vi "D - Level HWEng Port with Power Meter.vi"(5 "PM Ref":T1, 7 "Port (Port 3)":enum16{"Port 3", "Port 1(1)", "Port 1(2)"}(ring), 8 "error in (no error)":errorcluster, 9 "Frequency, MHz":dbl format="%.2f", 10 "Target Power, dBm":dbl format="%.2f") -> (0 "error out":errorcluster, 2 "Req'd Power \nfor Level, dBm":dbl, 3 "Actual Power at\nLevel, dBm":dbl)   [LabVIEW 2011]
uses:
  calibration/POWER METER/METER/Power Meter Object Reference.ctl
panel:
  out "No Tries":i32
  out "error":dbl
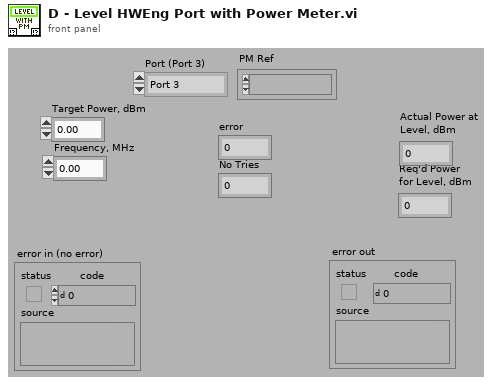
[diagram p1: front panel]
types:
  T1 = typedef "Power Meter Object Reference.ctl" = refnum<k1>
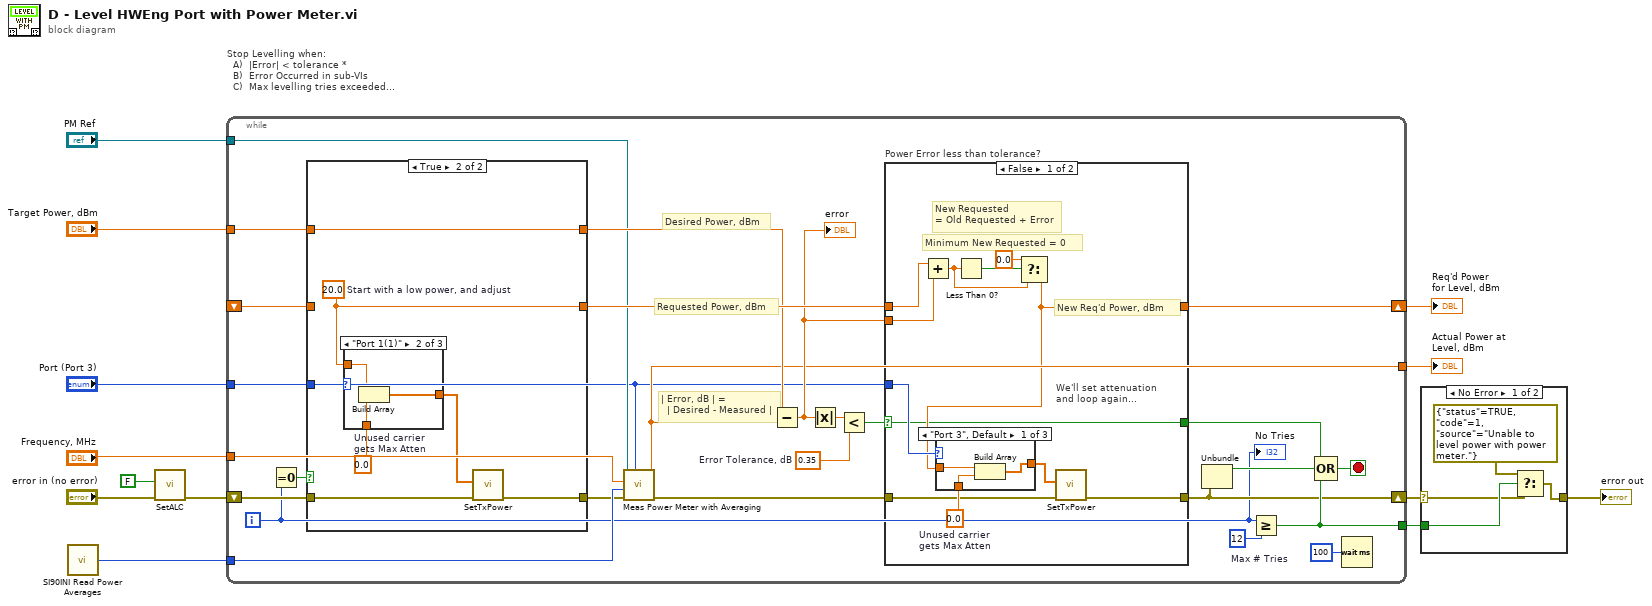
[diagram p0: block diagram]
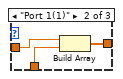
[diagram p2: hidden frame]
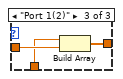
[diagram p3: hidden frame]
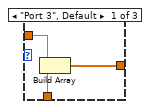
[diagram p6: hidden frame]
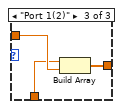
[diagram p7: hidden frame]
diagram:
  n1 = call "SI90INI Read Power Averages.vi"() -> ("Power Averages"=w4:i32)  [unwired: 5 in]
  n2 = call "SetALC.vi"("error in (no error)"="error in (no error)", "ALC"=FALSE) -> ("error out"=w2:errorcluster)  [unwired: 9 in]
  n3 = while "Stop Levelling when:\n  A)  |Error| < tolerance *\n  B)  Error Occurred in sub-VIs\n  C)  Max levelling tries exceeded\n\n* This is the only condition which gives NO ERROR" {
    tunnel: [w24] -> w10
    tunnel: "Frequency, MHz" -> [w26]
    tunnel: "Port (Port 3)" -> [w16]
    shift-left: _ -> [w32]
    shift-right: [w35] -> w6
    tunnel: "Target Power, dBm" -> [w30]
    shift-left: w2 -> [w19]
    shift-right: [w21] -> w12
    tunnel: "PM Ref" -> [w27]
    tunnel: [w23] -> w5
    tunnel: w4 -> [w25]
    i -> [w18]
    stop <- w36 stop-if-true
    w33 = 12  # Max # Tries
    w34 = 0.35  # Error Tolerance, dB
    # "Desired Power, dBm"
    # "| Error, dB | = \n  | Desired - Measured |"
    # "Requested Power, dBm"
    n4 = Equal To 0?(x=w18) -> (x = 0?=w17:bool)
    n5 = case shown="True" w17 {
      tunnel: w32 -> [w66 _]
      tunnel: [w66 w67] -> w31
      tunnel: w30 -> [w65 w68]
      tunnel: [w65 w68] -> w29
      tunnel: w19 -> [w64 w71]
      tunnel: w16 -> [_ w72]
      tunnel: [w64 w70] -> w15
      frame False {
      }
      frame True {
        w67 = 20.0  # Start with a low power, and adjust
        w73 = 0.0  # Unused carrier gets Max Atten
        n6 = case shown="\"Port 1(1)\"" w72 {
          tunnel: [w76 w79 w82] -> w69
          tunnel: w67 -> [w75 w78 w81]
          tunnel: w73 -> [w74 w77 w80]
          frame "Port 3", Default {
            n7 = Build Array(w75, w74) -> (w76:dbl[])
          }
          frame "Port 1(1)" {
            n8 = Build Array(w78, w77) -> (w79:dbl[])
          }
          frame "Port 1(2)" {
            n9 = Build Array(w80, w81) -> (w82:dbl[])
          }
        }
        n10 = call "SetTxPower.vi"("error in (no error)"=w71, "TxPower"=w69) -> ("error out"=w70:errorcluster)  [unwired: 9 in]
      }
    }
    n11 = call "Meas Power Meter with Averaging.vi"("Port (Port 3)"=w16, "error in (no error)"=w15, "Averages (1)"=w25, "Frequency, MHz"=w26, "PM Ref"=w27) -> ("error out"=w22:errorcluster, "Power, dBm"=w23:dbl)  [unwired: 4 in, 1 out]
    n12 = Subtract(x=w29, y=w23) -> (x-y=w28:dbl)
    "error" <- w28
    n13 = Absolute Value(x=w28) -> (abs(x)=w39:dbl)
    n14 = Less?(x=w39, y=w34) -> (x < y?=w20:bool)
    n15 = case "Power Error less than tolerance?" shown="False" w20 {
      selector: w20 -> [w43 w61]
      tunnel: [w44 w63] -> w35
      tunnel: w31 -> [w49 w63]
      tunnel: w28 -> [w48 _]
      tunnel: w22 -> [w42 w62]
      tunnel: [w41 w62] -> w21
      tunnel: w16 -> [w45 _]
      tunnel: [w43 w61] -> w14
      frame False {
        w46 = 0.0  # Unused carrier gets Max Atten
        # "We'll set attenuation\nand loop again..."
        # "New Req'd Power, dBm"
        # "New Requested\n= Old Requested + Error"
        # "Minimum New Requested = 0"
        n16 = Add(x=w49, y=w48) -> (x+y=w51:dbl)
        n17 = Less Than 0?(x=w51) -> (x < 0?=w47:bool)
        n18 = Select(t=0.0, s=w47, f=w51) -> (s? t:f=w44:dbl)
        n19 = case shown="\"Port 3\", Default" w45 {
          tunnel: [w54 w57 w60] -> w40
          tunnel: w44 -> [w53 w56 w59]
          tunnel: w46 -> [w52 w55 w58]
          frame "Port 3", Default {
            n20 = Build Array(w53, w52) -> (w54:dbl[])
          }
          frame "Port 1(1)" {
            n21 = Build Array(w56, w55) -> (w57:dbl[])
          }
          frame "Port 1(2)" {
            n22 = Build Array(w58, w59) -> (w60:dbl[])
          }
        }
        n23 = call "SetTxPower.vi"("error in (no error)"=w42, "TxPower"=w40) -> ("error out"=w41:errorcluster)  [unwired: 9 in]
      }
      frame True {
      }
    }
    n24 = Unbundle(w21) -> ("status"=w37:bool)  [unwired: 2 out]
    n25 = Greater Or Equal?(x=w18, y=w33) -> (x >= y?=w24:bool)
    n26 = Compound Arithmetic op=OR(w14, w37, w24) -> (w36:bool)
    n27 = Wait (ms)(milliseconds to wait=u32 100) -> ()  [unwired: 1 out]
    "No Tries" <- w18
  }
  "Req'd Power \nfor Level, dBm" <- w6
  "Actual Power at\nLevel, dBm" <- w5
  n28 = case shown="No Error" w12 {
    selector: w12 -> [w84 w87]
    tunnel: [w85 w87] -> w11
    tunnel: w10 -> [w86 _]
    frame No Error {
      n29 = Select(t=errorcluster {"status"=TRUE, "code"=1, "source"="Unable to level power with power meter."} ("error IO"), s=w86, f=w84) -> (s? t:f=w85:errorcluster)
    }
    frame Error {
    }
  }
  "error out" <- w11
